vi "SEA_CURRENT_CTL_PI_REF_TEST.vi"() -> ()   [LabVIEW 2019]
uses:
  <vilib>/Platform/TimedLoop/XDataNode/timing_clust.ctl
  <vilib>/Platform/TimedLoop/XDataNode/nitl_modes.ctl
  <vilib>/Platform/TimedLoop/XDataNode/wakeup.ctl
  <vilib>/FPGAPlugInAG/sbRIO-9627/niLvFpga_Open_sbRIO-9627.vi
  <vilib>/rvi/interface/common/dynamic/niFpgaDynamicAddResources.vi
  <vilib>/Utility/error.llb/Error Cluster From Error Code.vi
  <vilib>/rvi/errors/niLvFpgaAdjustHostInterfaceError.vi
  <vilib>/FPGAPlugInAG/Dynamic/niLvFpga_Close_Dynamic.vi
  <vilib>/rvi/interface/nirviOpenFPGA/nirviOpenFPGA.xnode
  FPGA Bitfiles/seafinalexperime_FPGATarget_SEALOWERLEVELPIC_AplcQzvwIw0.lvbitx
  SEA_LOWER_LEVEL_PI_CONTROL.vi
  <vilib>/Platform/TimedLoop/XDataNode/XDataNode.xnode
  <vilib>/rvi/interface/nirviReadWriteControl/nirviReadWriteControl.xnode
  <vilib>/rvi/interface/nirviCloseFPGA/nirviCloseFPGA.xnode
  <vilib>/Platform/TimedLoop/XDataNode/XDNodeRunTimeDep.lvlib
  NiFpgaLv.dll
  <vilib>/rvi/interface/Simulation/niFpgaSimulationCallBeginRW.vi
panel:
  in  "stop":bool
  out "Current":cluster{sgl, "filtered current":sgl}(graph)
  in  "Amplitude":sgl
  in  "frequency":sgl
  out "Loop rate":u32
  in  "Ki current control":sgl
  out "Motor Direction":bool
  in  "UB":sgl
  in  "LB":sgl
  in  "Current Offset":sgl
  in  "Kp current control":sgl
  out "Finished late count":u32
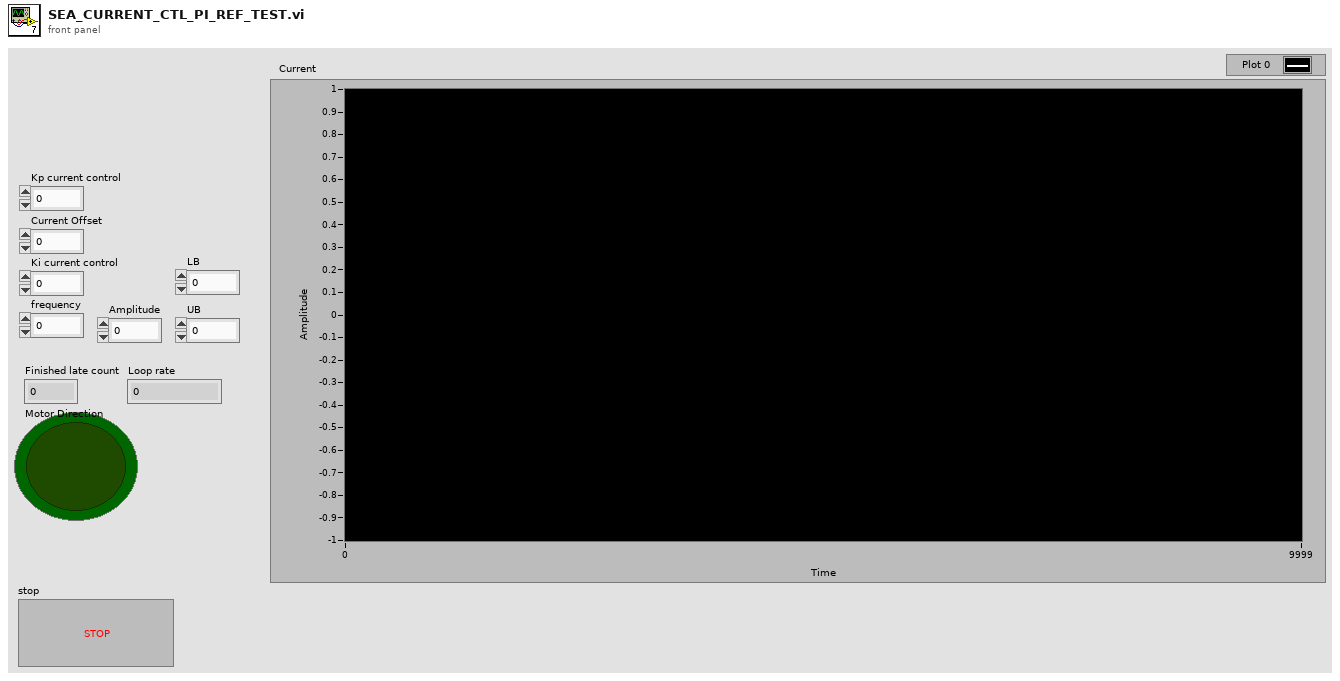
[diagram p1: front panel]
types:
  T1 = typedef "XDNodeRunTimeDep.lvlib/timing_clust.ctl" = cluster{"Expected End [f-1]":u64, "Actual End [f-1]":u64, "Finished Late? [f-1]":bool, "Expected End [i-1]":u64, "Actual End [i-1]":u64, "Finished Late? [i-1]":bool, "Expected Start [i]":u64, "Actual Start [i]":u64, "Expected Start [f]":u64, "Actual Start [f]":u64, "Source Name":string, "Structure Name":string, "Period":i64, "Deadline":i64, "Offset":i64, "Start":i64, "Priority":i32, "Timeout":i32, "Mode":T2, "Wakeup Reason":T3, "Error":errorcluster, "Source Type":string, "Secondary Source Type":string, "Global End Time":u64, "Global Start Time":u64, "Frame Duration":u64, "Iteration Duration":u64, "Assigned CPU":i32, "I/O Scan Engine Mode":u32}
  T2 = typedef "XDNodeRunTimeDep.lvlib/nitl_modes.ctl" = enum32{"No Change", "Process missed periods, maintain original phase", "Discard missed periods, maintain original phase", "Process missed periods, ignore original phase", "Discard missed periods, ignore original phase"}
  T3 = typedef "XDNodeRunTimeDep.lvlib/wakeup.ctl" = enum32{"Normal", "Aborted", "Asynchronous wakeup", "Timing source error", "Timed loop error", "Timeout"}
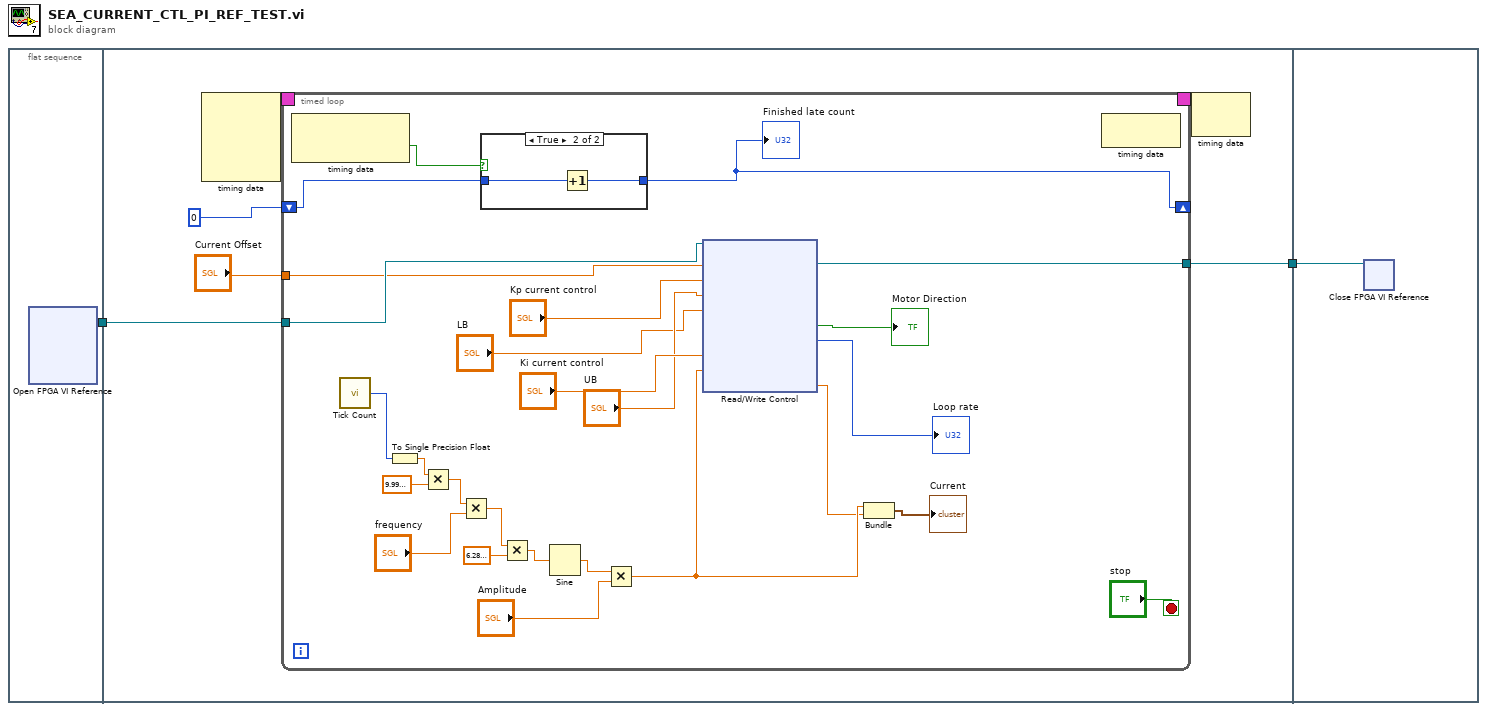
[diagram p0: block diagram]
diagram:
  n1 = flat-sequence {
    tunnel: [w3] -> w2
    tunnel: w2 -> [w6]
    tunnel: [w5] -> w1
    tunnel: w1 -> [w44]
    frame #0 {
      n2 = xnode "Open FPGA VI Reference"() -> ("FPGA VI Reference Out"=w3:refnum<k20>)  [unwired: 2 in, 1 out]
    }
    frame #1 {
      n3 = node-c288() -> (w9:T1)  [unwired: 4 in]
      n4 = timed-loop {
        timing: w9 -> [_]
        timing-out: [_] -> w8
        shift-right: [w33] -> _
        shift-left: u32 0 -> [w34]
        tunnel: w6 -> [w32]
        tunnel: [w31] -> w5
        tunnel: "Current Offset" -> [w10]
        stop <- "stop" stop-if-true
        n5 = node-c288() -> (w35:bool)  [unwired: 1 in, 1 out]
        n6 = call "Tick Count"() -> ("Tick Count(uSec)"=w26:u32)
        n7 = To Single Precision Float(number=w26) -> (single precision float=w25:sgl)
        n8 = Multiply(x=w25, y=sgl 1e-06) -> (x*y=w23:sgl)
        n9 = Multiply(x=w23, y="frequency") -> (x*y=w21:sgl)
        n10 = case shown="True" w35 {
          tunnel: w34 -> [w36 w38]
          tunnel: [w36 w37] -> w33
          frame False {
          }
          frame True {
            n11 = Increment(x=w38) -> (x+1=w37:u32)
          }
        }
        "Finished late count" <- w33
        n12 = Multiply(x=w21, y=sgl 6.28) -> (x*y=w19:sgl)
        n13 = Sine(x=w19) -> (sin(x)=w18:sgl)
        n14 = Multiply(x=w18, y="Amplitude") -> (x*y=w16:sgl)
        n15 = xnode "Read/Write Control"("FPGA VI Reference In"=w32, "Current Offset"=w10, "Kp current control"="Kp current control", "Upper bound"="UB", "Lower bound"="LB", "Ki current control"="Ki current control", "Reference"=w16) -> ("FPGA VI Reference Out"=w31:refnum<k20>, "Motor direction"=→"Motor Direction":bool, "Loop rate"=→"Loop rate":u32, "filtered current"=w15:sgl)  [unwired: 1 in, 1 out]
        n16 = Bundle(w16, "filtered current"=w15) -> (→"Current":cluster{sgl, "filtered current":sgl})  [unwired: 1 in]
        n17 = node-c288() -> ()  [unwired: 1 in, 1 out]
      }
      n18 = node-c288(w8) -> ()  [unwired: 1 out]
    }
    frame #2 {
      n19 = xnode "Close FPGA VI Reference"("FPGA VI Reference In"=w44) -> ()  [unwired: 1 in, 1 out]
    }
  }
